vi "OTA Test 1.vi"(8 "Error In":errorcluster) -> (0 "Error Out":errorcluster)   [LabVIEW 2014, in "ESP8266 WiFi Wrapper.lvlib"]
uses:
  ESP8266 WiFi Wrapper.lvlib
  utils/OTA Blink LED.vi
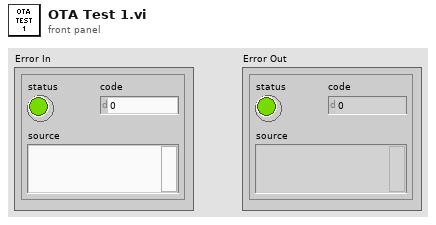
[diagram p1: front panel]
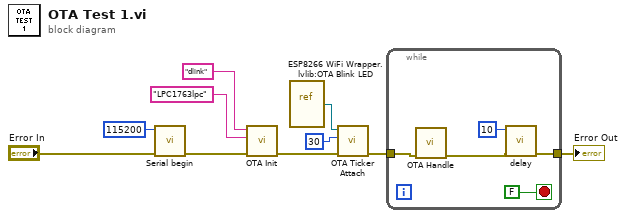
[diagram p0: block diagram]
diagram:
  n1 = call <vilib>:"Serial begin.vi"("Error In"="Error In", "speed (Bd)"=115200) -> ("Error Out"=w8:errorcluster)  [unwired: 9 in]
  n2 = call "OTA Init.vi"("Error In"=w8, "password"="LPC1763lpc" ("ssid"), "ssid"="dlink") -> ("Error Out"=w5:errorcluster)  [unwired: 8 in]
  n3 = vi-ref "ESP8266 WiFi Wrapper.lvlib:OTA Blink LED.vi"() -> (w4:refnum<vi>)
  n4 = call "OTA Ticker Attach.vi"("Error In"=w5, "interval (sec.)"=u32 30, "VI Refnum"=w4) -> ("Error Out"=w2:errorcluster)  [unwired: 8 in]
  n5 = while {
    tunnel: w2 -> [w15]
    tunnel: [w12] -> w3
    stop <- FALSE stop-if-true
    n6 = call "OTA Handle.vi"("Error In"=w15) -> ("Error Out"=w13:errorcluster)  [unwired: 10 in]
    n7 = call <vilib>:"delay.vi"("Error In"=w13, "time (ms)"=10) -> ("Error Out"=w12:errorcluster)  [unwired: 9 in]
  }
  "Error Out" <- w3
